vi "Get_Tims.vi"(8 "error in (no error)":errorcluster caption="错误输入（无错误）") -> (0 "error out":errorcluster caption="错误输出", 2 "连接的字符串":string)   [LabVIEW 2018]
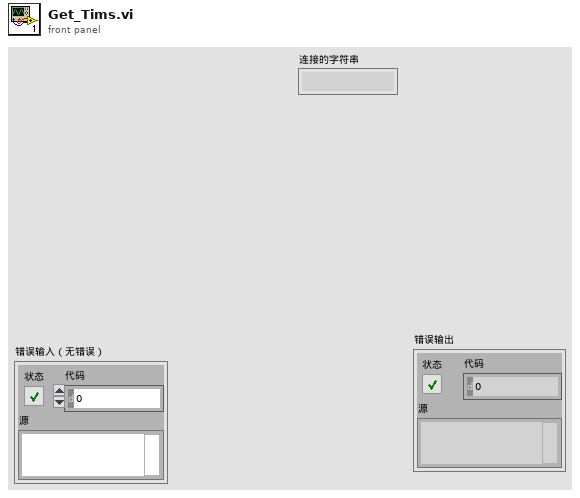
[diagram p1: front panel]
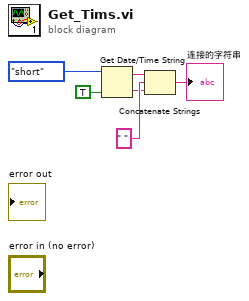
[diagram p0: block diagram]
diagram:
  n1 = Get Date/Time String(date format (0)=enum16{"short", "long", "abbreviated"}."short" ("日期格式(0)"), want seconds? (F)=TRUE ("需要秒？(F)")) -> (date string=w6:string, time string=w4:string)  [unwired: 1 in]
  n2 = Concatenate Strings(w6, " ", w4) -> (→"连接的字符串":string)
